vi "Execute.UI.Complete.vi"(8 "error in (no error)":errorcluster, 11 "Cluster":T1={"NIVS.BaseLogPath"=path "", "NIVS.SystemDefinitionFile"=path "", "NIVS.Events"={"SequenceEvent"=refnum, "SystemChangeEvent"=refnum, "WorkspaceEvent"=refnum}, "NIVS.SequenceState"=enum."Idle", "NIVS.GatewayIPAddress"="", "NIVS.DataLogSpecRef"=refnum, "NIVS.DataLogManagerRef"=refnum, "NIVS.LogSessionGUID"="", "NIVS.WorkspaceManager"=refnum, "NIVS.Deployed"=FALSE, "NIVS.ProfileRef"=refnum, "NIVS.ProfileCallback"=refnum, "NIVS.SystemStateRefs"={"CustDatRef"=refnum, "EvtRef"=refnum}, "UI.Abort"=refnum, "UI.Pause"=refnum, "UI.EnableLogging"=refnum, "UI.Start"=refnum, "UI.LogChannels"=refnum, "UI.StartIteration"=refnum, "UI.StartStep"=refnum, "UI.Sequence"=refnum, "UI.PreviewMode"=refnum, "UI.Graph"=refnum, "UI.BaseFileName"=refnum, "UI.Profiles"=refnum, "UI.CurrentStep"=refnum, "UI.CurrentIteration"=refnum, "UI.TotalIterations"=refnum, "Sequence.AbortChannel"="", "Sequence.StepInfoChannel"="", "Sequence.Iterations"=0, "Sequence.IterationInfoChannel"="", "Sequence.#ofColumns"=0, "Events.State"=refnum, "Events.Test Result"=refnum, "Events.Progress"=refnum, "INI.Settings"={"Build Location"=path "C:/Simple Sequence Editor/SequenceRepo", "LoggingLocation"=path ""}}) -> (0 "error out":errorcluster)   [LabVIEW 2013, in "Simple Sequence Tools - Execution.lvlib"]
uses:
  Simple Sequence Tools - Execution.lvlib
  Types/Main.StateVariables.ctl
  Types/Execute.UserEventRefs.ctl
  <vilib>/NI Veristand/Execution/Workspace/SystemStateRegEventRef.ctl
  Types/Execution.SequenceState.ctl
  <vilib>/NI Veristand/Execution/DataLogging/DataLoggingSpecification Ref.ctl
  NationalInstruments.VeriStand.ClientAPI
  <vilib>/NI Veristand/Execution/DataLogging/IDataLogging Ref.ctl
  <vilib>/NI Veristand/Execution/Workspace/WorkspaceAPI.ctl
  NationalInstruments.VeriStand.RealTimeSequenceDefinitionApi
  <vilib>/NI Veristand/Execution/Workspace/SystemStateEventRef.ctl
  Shared/Types/INI.Settings
  <vilib>/NI Veristand/Execution/Workspace/NI_VS Workspace ExecutionAPI.lvlib
  <vilib>/NI Veristand/Execution/DataLogging/NI_VS Data Logging API.lvlib
  Shared/Simple Sequence Tools - Shared.lvlib
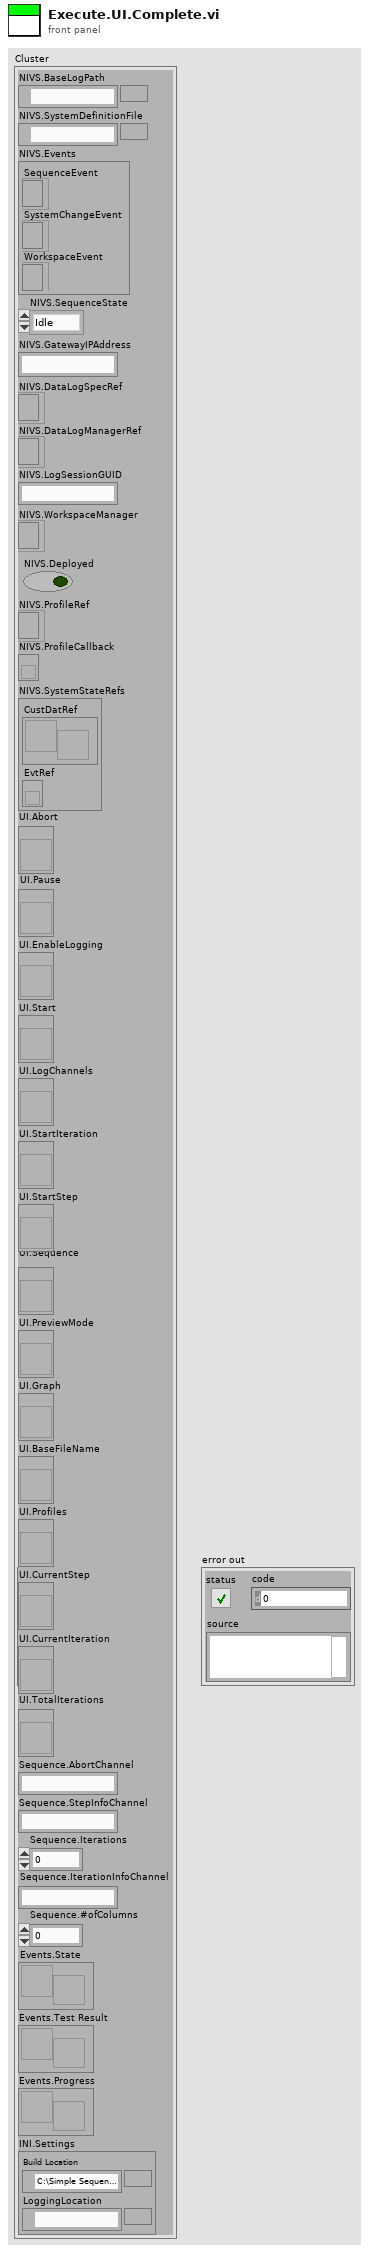
[diagram p1: front panel]
types:
  T1 = typedef "Simple Sequence Tools - Execution.lvlib/Main.StateVariables.ctl" = cluster{"NIVS.BaseLogPath":path, "NIVS.SystemDefinitionFile":path, "NIVS.Events":T2, "NIVS.SequenceState":T4, "NIVS.GatewayIPAddress":string, "NIVS.DataLogSpecRef":T5, "NIVS.DataLogManagerRef":T6, "NIVS.LogSessionGUID":string, "NIVS.WorkspaceManager":T7, "NIVS.Deployed":bool, "NIVS.ProfileRef":refnum<k24>, "NIVS.ProfileCallback":refnum<k27>, "NIVS.SystemStateRefs":T8, "UI.Abort":refnum<vi>, "UI.Pause":refnum<vi>, "UI.EnableLogging":refnum<vi>, "UI.Start":refnum<vi>, "UI.LogChannels":refnum<vi>, "UI.StartIteration":refnum<vi>, "UI.StartStep":refnum<vi>, "UI.Sequence":refnum<vi>, "UI.PreviewMode":refnum<vi>, "UI.Graph":refnum<vi>, "UI.BaseFileName":refnum<vi>, "UI.Profiles":refnum<vi>, "UI.CurrentStep":refnum<vi>, "UI.CurrentIteration":refnum<vi>, "UI.TotalIterations":refnum<vi>, "Sequence.AbortChannel":string, "Sequence.StepInfoChannel":string, "Sequence.Iterations":u32, "Sequence.IterationInfoChannel":string, "Sequence.#ofColumns":i32, "Events.State":refnum<user-event>, "Events.Test Result":refnum<user-event>, "Events.Progress":refnum<user-event>, "INI.Settings":T9}
  T2 = typedef "Simple Sequence Tools - Execution.lvlib/Execute.UserEventRefs.ctl" = cluster{"SequenceEvent":refnum<event-registration>, "SystemChangeEvent":T3, "WorkspaceEvent":refnum<event-registration>}
  T3 = typedef "NI_VS Workspace ExecutionAPI.lvlib/SystemStateRegEventRef.ctl" = refnum<event-registration>
  T4 = typedef "Simple Sequence Tools - Execution.lvlib/Execution.SequenceState.ctl" = enum16{"Idle", "Initializing", "Running", "Paused", "Finalizing", "Complete"}
  T5 = typedef "NI_VS Data Logging API.lvlib/DataLoggingSpecification Ref.ctl" = refnum<k24>
  T6 = typedef "NI_VS Data Logging API.lvlib/IDataLogging Ref.ctl" = refnum<k24>
  T7 = typedef "NI_VS Workspace ExecutionAPI.lvlib/WorkspaceAPI.ctl" = refnum<k24>
  T8 = typedef "NI_VS Workspace ExecutionAPI.lvlib/SystemStateEventRef.ctl" = cluster{"CustDatRef":refnum<user-event>, "EvtRef":refnum<k27>}
  T9 = typedef "Simple Sequence Tools - Shared.lvlib/INI.Settings" = cluster{"Build Location":path, "LoggingLocation":path}
  T10 = enum8{"Enabled", "Disabled", "Disabled and Grayed Out"}
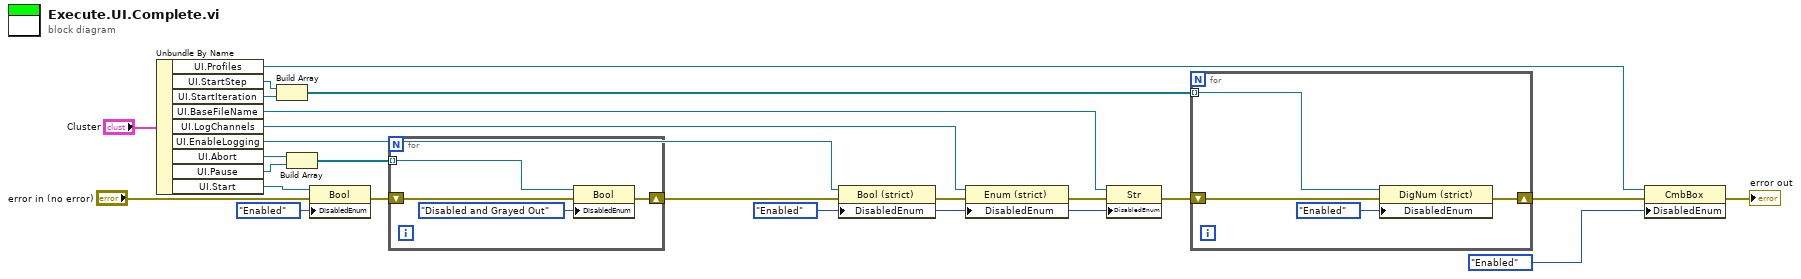
[diagram p0: block diagram]
diagram:
  w5 = T10."Enabled" ("Disabled")
  n1 = Unbundle By Name("Cluster") -> ("UI.Profiles"=w23:refnum<vi>, "UI.StartStep"=w20:refnum<vi>, "UI.StartIteration"=w19:refnum<vi>, "UI.BaseFileName"=w6:refnum<vi>, "UI.LogChannels"=w17:refnum<vi>, "UI.EnableLogging"=w16:refnum<vi>, "UI.Abort"=w12:refnum<vi>, "UI.Pause"=w13:refnum<vi>, "UI.Start"=w7:refnum<vi>)
  n2 = Build Array(w20, w19) -> (w21:refnum<vi>[])
  n3 = Build Array(w12, w13) -> (w14:refnum<vi>[])
  n4 = property class="Bool"(reference=w7, error in="error in (no error)", "DisabledEnum"=T10."Enabled" ("Disabled")) -> (error out=w8:errorcluster)  [unwired: 1 out]
  n5 = for {
    tunnel: w14 -> [w27] mode=indexing
    shift-right: [w25] -> w15
    shift-left: w8 -> [w24]
    n6 = property class="Bool"(reference=w27, error in=w24, "DisabledEnum"=T10."Disabled and Grayed Out" ("Disabled")) -> (error out=w25:errorcluster)  [unwired: 1 out]
  }
  n7 = property class="Bool (strict)"(reference=w16, error in=w15, "DisabledEnum"=w5) -> (error out=w18:errorcluster)  [unwired: 1 out]
  n8 = property class="Enum (strict)"(reference=w17, error in=w18, "DisabledEnum"=w5) -> (error out=w4:errorcluster)  [unwired: 1 out]
  n9 = property class="Str"(reference=w6, error in=w4, "DisabledEnum"=w5) -> (error out=w3:errorcluster)  [unwired: 1 out]
  n10 = for {
    tunnel: w21 -> [w31] mode=indexing
    shift-right: [w29] -> w22
    shift-left: w3 -> [w28]
    n11 = property class="DigNum (strict)"(reference=w31, error in=w28, "DisabledEnum"=T10."Enabled" ("Disabled")) -> (error out=w29:errorcluster)  [unwired: 1 out]
  }
  n12 = property class="CmbBox"(reference=w23, error in=w22, "DisabledEnum"=T10."Enabled" ("Disabled")) -> (error out=→"error out":errorcluster)  [unwired: 1 out]
